vi "_N-MarkdownTitle.vi"(11 "Numeric":i32) -> (3 "String":string)   [LabVIEW 2017, in "csmdoc.lvlib"]
uses:
  csmdoc.lvlib
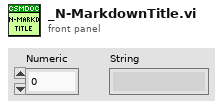
[diagram p1: front panel]
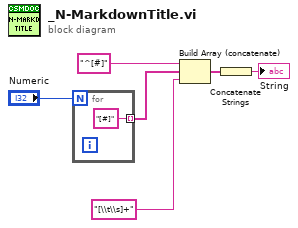
[diagram p0: block diagram]
diagram:
  n1 = for {
    N: "Numeric" -> [_]
    tunnel: ["[#]" ("delimited string")] -> w3 mode=indexing
  }
  n2 = Build Array (concatenate)("^[#]" ("delimited string"), w3, "[\\t\\s]+" ("delimited string")) -> (w1:string[])
  n3 = Concatenate Strings(w1) -> (→"String":string)
